vi "img.Percentile.vi"(10 "U16 image in":u16[][](array[numeric])) -> (2 "U32 image out":u32[][](array[numeric]))   [LabVIEW 2020]
uses:
  _controls/perc.ctl
  pix.sgl.CalcPercentiles.vi
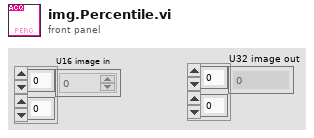
[diagram p1: front panel]
types:
  T1 = typedef "perc.ctl" = enum16{"0-100%", "1-99%", "5-95%", "10-90%", "20-80%"}
  T2 = typedef "cluster.range.sgl.ctl" = cluster{"min":sgl, "max":sgl}
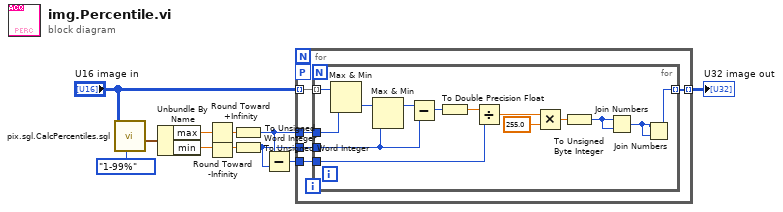
[diagram p0: block diagram]
diagram:
  n1 = call "pix.sgl.CalcPercentiles.sgl.vi"("percentiles"=perc."1-99%", "img in"="U16 image in") -> ("range"=w9:T2)  [unwired: 9 in]
  n2 = Unbundle By Name(w9) -> ("max"=w5:sgl, "min"=w8:sgl)
  n3 = Round Toward +Infinity(x=w5) -> (ceil(x): smallest int >= x=w7:sgl)
  n4 = Round Toward -Infinity(1:w8) -> (0:w6:sgl)
  n5 = To Unsigned Word Integer(number=w7) -> (unsigned 16bit integer=w3:u16)
  n6 = To Unsigned Word Integer(number=w6) -> (unsigned 16bit integer=w2:u16)
  n7 = Subtract(x=w3, y=w2) -> (x-y=w1:u16)
  n8 = for {
    tunnel: "U16 image in" -> [w16] mode=indexing
    tunnel: w2 -> [w15]
    tunnel: w3 -> [w14]
    workers-P: _ -> [_]
    tunnel: [w13] -> w4 mode=indexing
    tunnel: w1 -> [w12]
    n9 = for {
      tunnel: w16 -> [w30] mode=indexing
      tunnel: [w23] -> w13 mode=indexing
      tunnel: w14 -> [w24]
      tunnel: w15 -> [w17]
      tunnel: w12 -> [w21]
      n10 = Max & Min(x=w30, y=w24) -> (min(x,y)=w20:u16)  [unwired: 1 out]
      n11 = Max & Min(x=w20, y=w17) -> (max(x,y)=w19:u16)  [unwired: 1 out]
      n12 = Subtract(x=w19, y=w17) -> (x-y=w18:u16)
      n13 = To Double Precision Float(number=w18) -> (double precision float=w29:dbl)
      n14 = Divide(x=w29, y=w21) -> (x/y=w28:dbl)
      n15 = Multiply(x=w28, y=255.0) -> (x*y=w22:dbl)
      n16 = To Unsigned Byte Integer(number=w22) -> (unsigned 8bit integer=w26:u8)
      n17 = Join Numbers(hi=w26, lo=w26) -> ((hi.lo)=w25:u16)
      n18 = Join Numbers(hi=w25, lo=w25) -> ((hi.lo)=w23:u32)
    }
  }
  "U32 image out" <- w4
